vi "Boiler.vi"(8 "error in":errorcluster, 9 "Boiler Configuration":T2, 10 "Notifiers":T1, 11 "Message Queues":T3) -> (0 "error out":errorcluster)   [LabVIEW 2015, in "Boiler.lvlib"]
doc: "This module simulates the behavior of a boiler. It receives a command from the boiler controller, executes, and then notifies the boiler controller that it has completed the operation."
uses:
  Boiler.lvlib
  support/Message Queue/All Message Queues.ctl
  support/Message Queue/Message Cluster.ctl
  Boiler Configuration.ctl
  support/Notifiers/Notifiers.ctl
  Boiler Data.ctl
  Boiler UI Data.ctl
  Boiler References.ctl
  <vilib>/Utility/error.llb/Error Cluster From Error Code.vi
  <vilib>/ErrorRing/Error Ring.xnode
  support/Message Queue/Message Queue.lvlib
panel:
  out "Pilot Flame Level (%)":u32(knob) scale=0.0..100.0
  out "Fuel Level (%)":u32(slide) scale=0.0..100.0
  in  "Simulate Failure":bool
  out "Forced Draft Fan":bool
  out "Pilot":bool
  out "Pilot Gas":bool
  out "Primary Fan":bool
  out "Run Interlock":bool
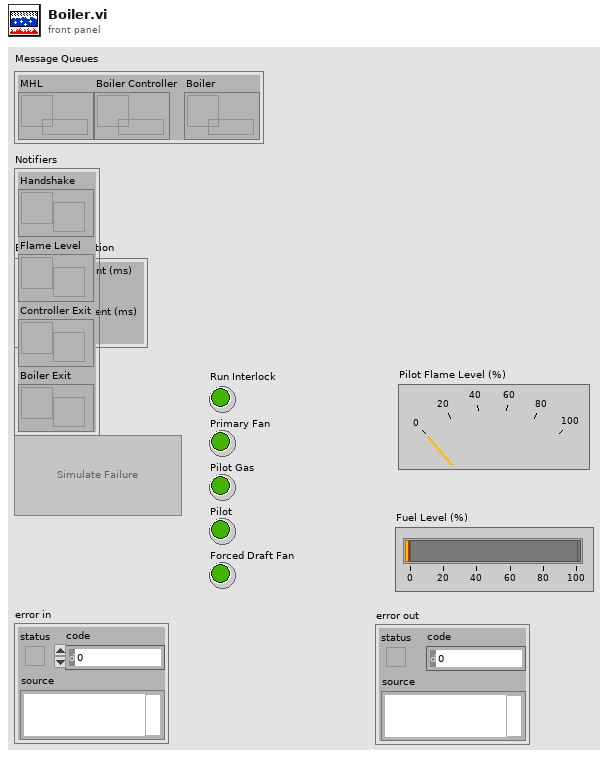
[diagram p1: front panel]
types:
  T1 = typedef "Notifiers.ctl" = cluster{"Handshake":refnum<notifier>, "Flame Level":refnum<notifier>, "Controller Exit":refnum<notifier>, "Boiler Exit":refnum<notifier>}
  T2 = typedef "Boiler.lvlib/Boiler Configuration.ctl" = cluster{"Pilot Increment (ms)":u32, "Pilot Decrement (ms)":u32}
  T3 = typedef "Message Queue.lvlib/All Message Queues.ctl" = cluster{"MHL":refnum<queue>, "Boiler Controller":refnum<queue>, "Boiler":refnum<queue>}
  T4 = typedef "Boiler.lvlib/Boiler Data.ctl" = cluster{"Boiler User Interface Data":T5, "Boiler Configuration":T2, "Boiler References":T6}
  T5 = typedef "Boiler.lvlib/Boiler UI Data.ctl" = cluster{"Run Interlock":bool, "Primary Fan":bool, "Pilot Gas":bool, "Pilot":bool, "Forced Draft Fan":bool, "Pilot Flame Level (%)":u32, "Boiler Flame Level (%)":u32}
  T6 = typedef "Boiler.lvlib/Boiler References.ctl" = cluster{"Simulate Failure":refnum<vi>}
  T7 = enum8{"Enabled", "Disabled", "Disabled and Grayed Out"}
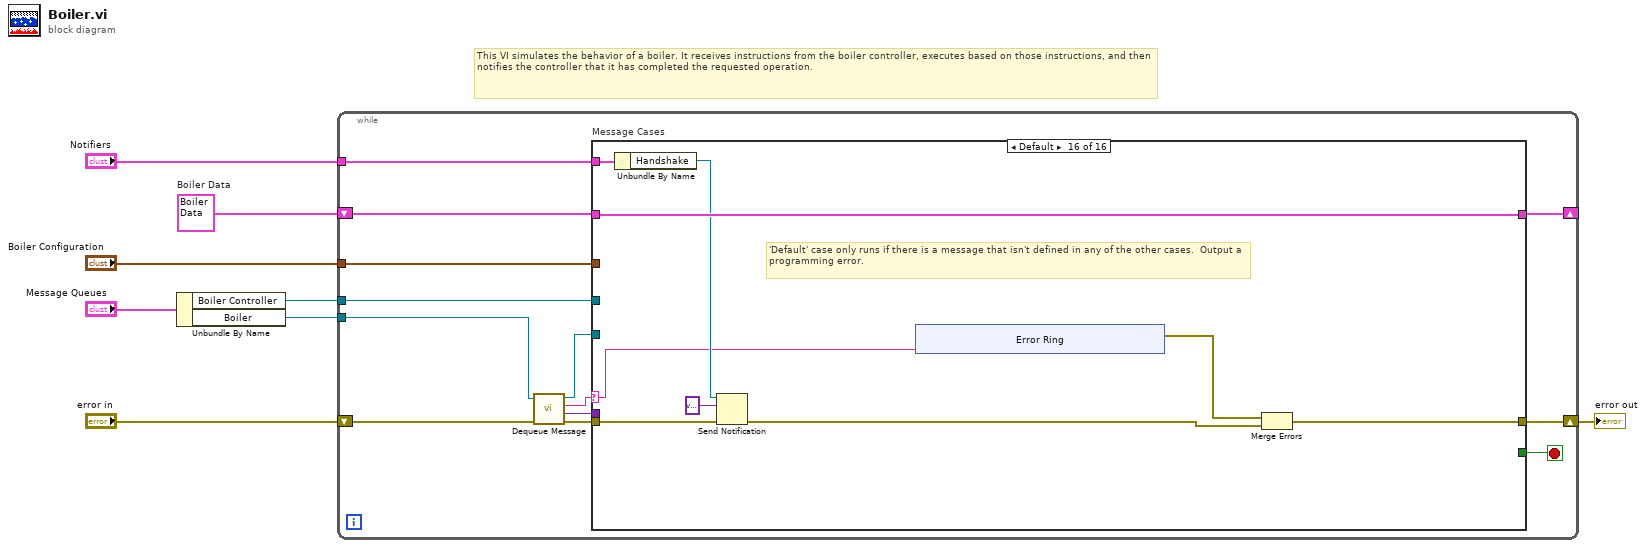
[diagram p0: block diagram]
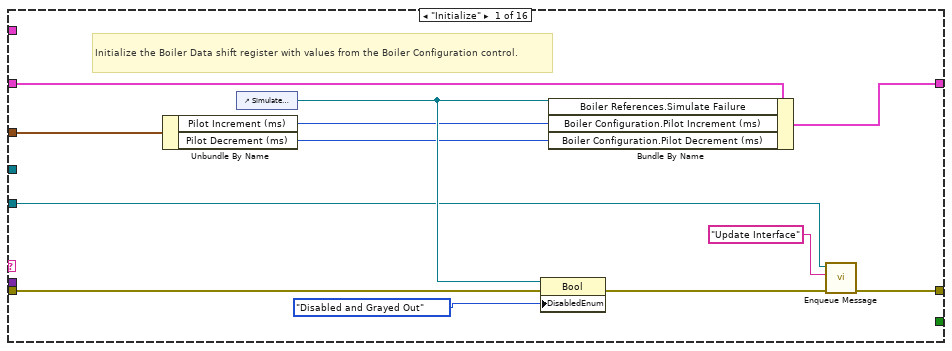
[diagram p2: hidden frame]
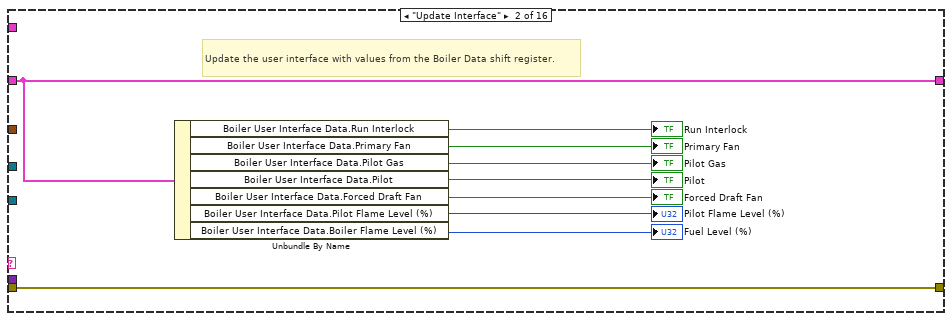
[diagram p3: hidden frame]
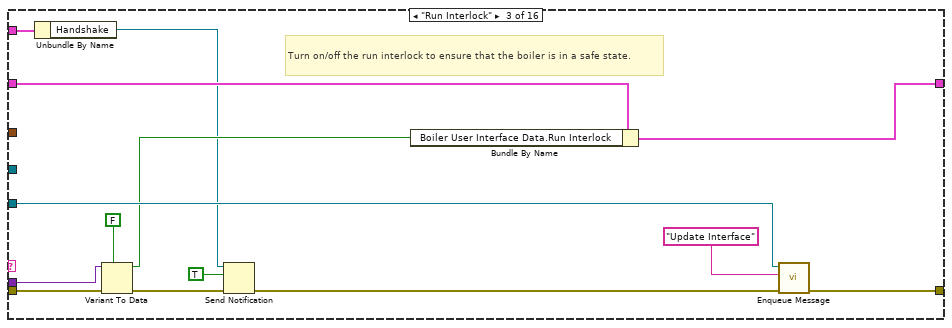
[diagram p4: hidden frame]
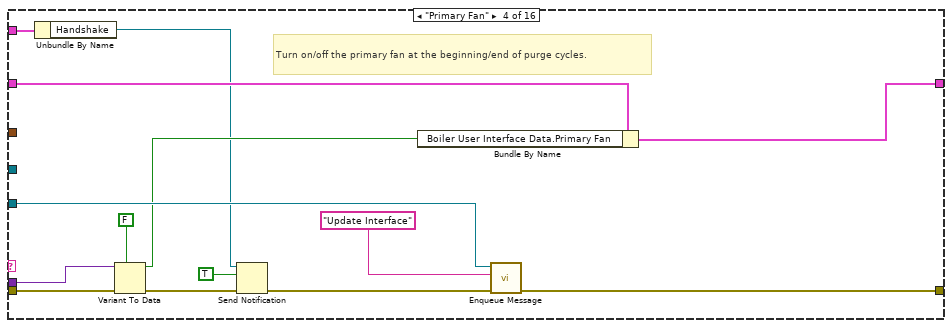
[diagram p5: hidden frame]
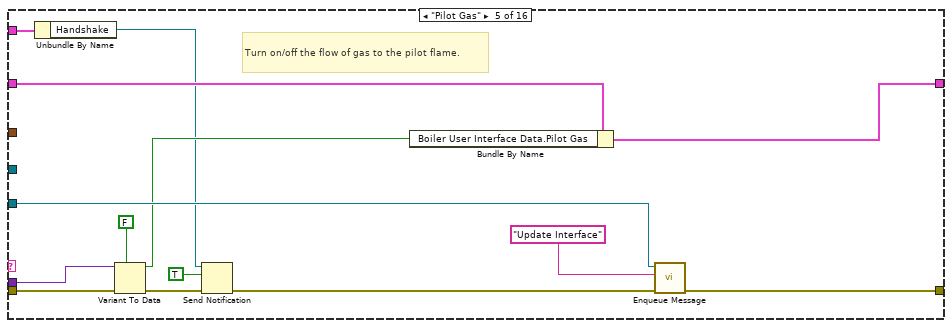
[diagram p6: hidden frame]
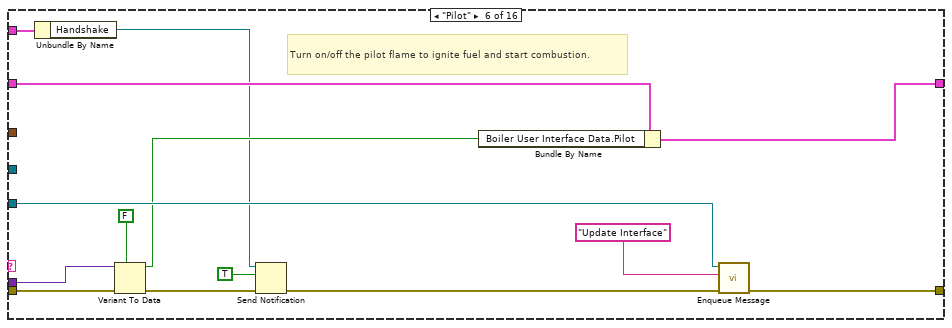
[diagram p7: hidden frame]
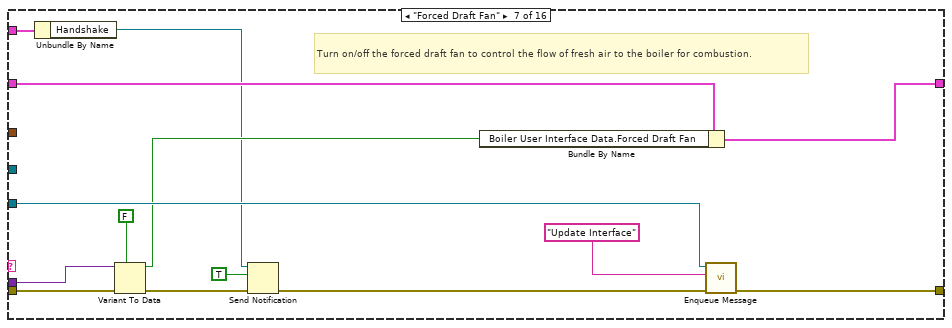
[diagram p8: hidden frame]
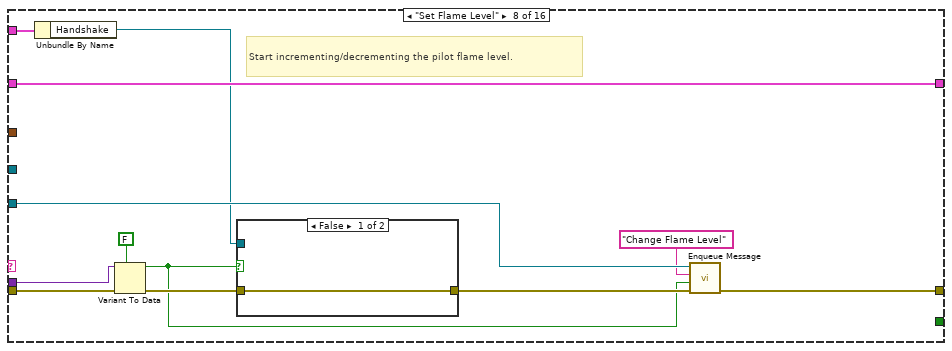
[diagram p9: hidden frame]
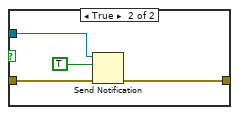
[diagram p10: hidden frame]
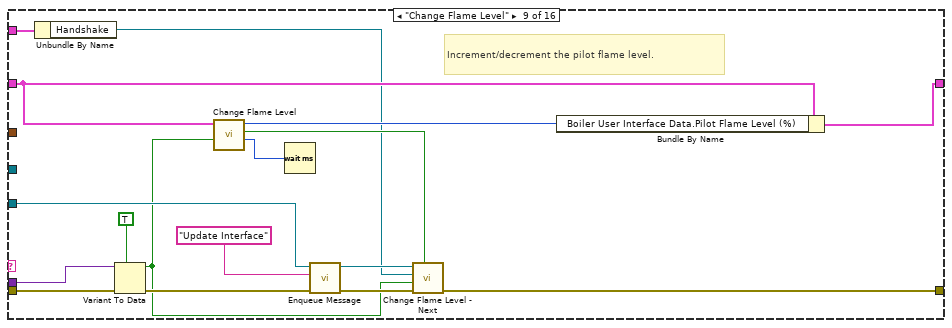
[diagram p11: hidden frame]
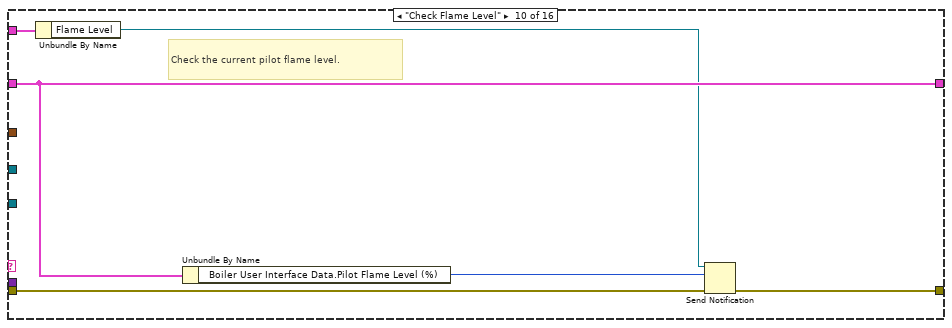
[diagram p12: hidden frame]
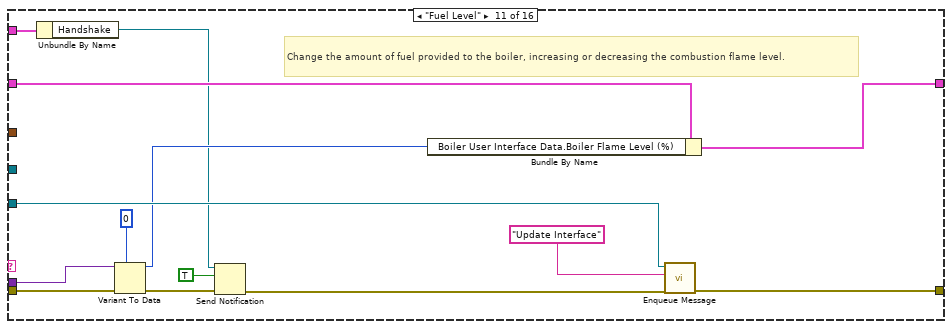
[diagram p13: hidden frame]
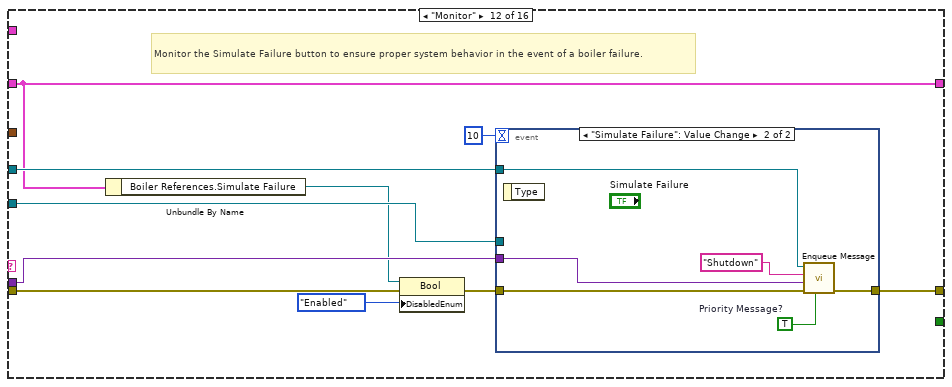
[diagram p14: hidden frame]
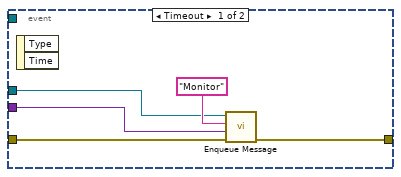
[diagram p15: hidden frame]
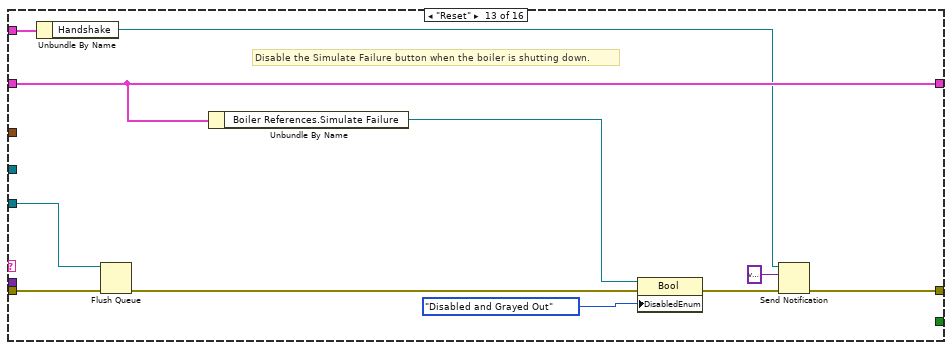
[diagram p16: hidden frame]
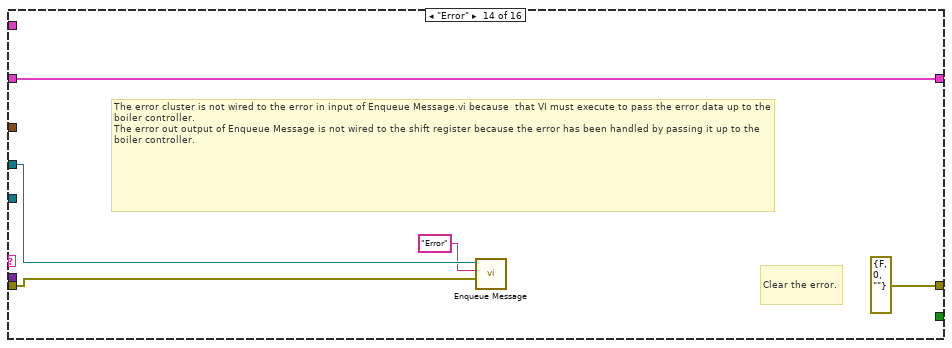
[diagram p17: hidden frame]
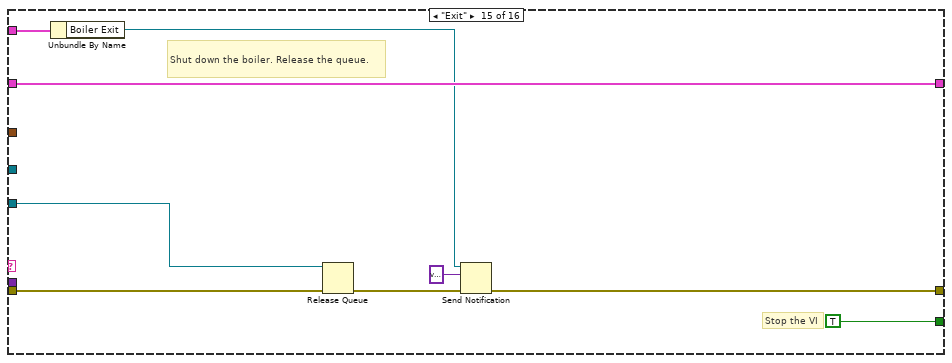
[diagram p18: hidden frame]
diagram:
  w7 = T4 {"Boiler User Interface Data"={"Run Interlock"=FALSE, "Primary Fan"=FALSE, "Pilot Gas"=FALSE, "Pilot"=FALSE, "Forced Draft Fan"=FALSE, "Pilot Flame Level (%)"=0, "Boiler Flame Level (%)"=0}, "Boiler Configuration"={"Pilot Increment (ms)"=0, "Pilot Decrement (ms)"=0}, "Boiler References"={"Simulate Failure"=refnum}}  # Boiler Data
  # "This VI simulates the behavior of a boiler. It receives instructions from the boiler controller, executes based on those instructions, and then notifies the controller that it has completed the requested operation."
  n1 = Unbundle By Name("Message Queues") -> ("Boiler Controller"=w4:refnum<queue>, "Boiler"=w3:refnum<queue>)
  n2 = while {
    tunnel: w3 -> [w12]
    shift-right: [w20] -> _
    shift-left: w7 -> [w21]
    shift-right: [w18] -> w8
    shift-left: "error in" -> [w17]
    tunnel: w4 -> [w11]
    tunnel: "Notifiers" -> [w10]
    tunnel: "Boiler Configuration" -> [w9]
    stop <- w19 stop-if-true
    n3 = call "Dequeue Message.vi"("error in (no error)"=w17, "Message Queue"=w12) -> ("error out"=w16:errorcluster, "Message Data"=w14:variant, "Message"=w15:string, "dup Message Queue"=w13:refnum<queue>)  [unwired: 6 in]
    n4 = case "Message Cases" shown="Default" w15 {
      selector: w15 -> [_ _ _ _ _ _ _ _ _ _ _ _ _ _ _ w213]
      tunnel: w13 -> [w27 _ w56 w66 w80 w94 w108 w122 w143 _ w163 w175 w195 _ w212 _]
      tunnel: w16 -> [w23 w36 w55 w68 w82 w96 w110 w119 w145 w149 w165 w167 w194 w200 w209 w220]
      tunnel: [w28 w36 w47 w60 w74 w88 w102 w123 w134 w152 w156 w168 w192 errorcluster {"status"=FALSE, "code"=0, "source"=""} ("error out") w208 w219] -> w18
      tunnel: w21 -> [w31 w42 w52 w65 w79 w93 w107 w124 w142 w151 w161 w169 w197 w203 w211 w221]
      tunnel: [w32 w42 w49 w64 w78 w92 w105 w124 w141 w151 w159 w169 w197 w203 w211 w221] -> w20
      tunnel: [_ _ _ _ _ _ _ _ _ _ _ _ _ _ TRUE _] -> w19
      tunnel: w14 -> [_ _ w53 w67 w81 w95 w109 w118 w144 _ w164 w173 _ _ _ _]
      tunnel: w11 -> [_ _ _ _ _ _ _ _ _ _ _ w174 _ w202 _ _]
      tunnel: w10 -> [_ _ w45 w59 w73 w87 w101 w114 w133 w150 w155 _ w191 _ w207 w217]
      tunnel: w9 -> [w26 _ _ _ _ _ _ _ _ _ _ _ _ _ _ _]
      frame "Initialize" {
        # "Initialize the Boiler Data shift register with values from the Boiler Configuration control."
        n5 = Unbundle By Name(w26) -> ("Pilot Increment (ms)"=w25:u32, "Pilot Decrement (ms)"=w24:u32)
        n6 = control-ref of="Simulate Failure"() -> (w30:refnum<vi>)
        n7 = property class="Bool"(reference=w30, error in=w23, "DisabledEnum"=T7."Disabled and Grayed Out" ("Disabled")) -> (error out=w22:errorcluster)  [unwired: 1 out]
        n8 = Bundle By Name(cluster=w31, "Boiler References.Simulate Failure"=w30, "Boiler Configuration.Pilot Increment (ms)"=w25, "Boiler Configuration.Pilot Decrement (ms)"=w24) -> (w32:T4)
        n9 = call "Enqueue Message.vi"("error in (no error)"=w22, "Message"="Update Interface", "Message Queue"=w27) -> ("error out"=w28:errorcluster)  [unwired: 7 in, 1 out]
      }
      frame "Update Interface" {
        # "Update the user interface with values from the Boiler Data shift register."
        n10 = Unbundle By Name(w42) -> ("Boiler User Interface Data.Run Interlock"=→"Run Interlock":bool, "Boiler User Interface Data.Primary Fan"=→"Primary Fan":bool, "Boiler User Interface Data.Pilot Gas"=→"Pilot Gas":bool, "Boiler User Interface Data.Pilot"=→"Pilot":bool, "Boiler User Interface Data.Forced Draft Fan"=→"Forced Draft Fan":bool, "Boiler User Interface Data.Pilot Flame Level (%)"=→"Pilot Flame Level (%)":u32, "Boiler User Interface Data.Boiler Flame Level (%)"=→"Fuel Level (%)":u32)
      }
      frame "Run Interlock" {
        # "Turn on/off the run interlock to ensure that the boiler is in a safe state."
        n11 = Unbundle By Name(w45) -> ("Handshake"=w43:refnum<notifier>)
        n12 = Variant To Data(error in=w55, type=FALSE ("Run Interlock"), Variant=w53) -> (data=w51:bool, error out=w48:errorcluster)
        n13 = Send Notification(notification=TRUE, notifier=w43, error in (no error)=w48) -> (error out=w46:errorcluster)  [unwired: 1 out]
        n14 = Bundle By Name(cluster=w52, "Boiler User Interface Data.Run Interlock"=w51) -> (w49:T4)
        n15 = call "Enqueue Message.vi"("error in (no error)"=w46, "Message"="Update Interface", "Message Queue"=w56) -> ("error out"=w47:errorcluster)  [unwired: 7 in, 1 out]
      }
      frame "Primary Fan" {
        # "Turn on/off the primary fan at the beginning/end of purge cycles."
        n16 = Unbundle By Name(w59) -> ("Handshake"=w57:refnum<notifier>)
        n17 = Variant To Data(error in=w68, type=FALSE ("Run Interlock"), Variant=w67) -> (data=w63:bool, error out=w62:errorcluster)
        n18 = Send Notification(notification=TRUE ("Run Interlock"), notifier=w57, error in (no error)=w62) -> (error out=w61:errorcluster)  [unwired: 1 out]
        n19 = Bundle By Name(cluster=w65, "Boiler User Interface Data.Primary Fan"=w63) -> (w64:T4)
        n20 = call "Enqueue Message.vi"("error in (no error)"=w61, "Message"="Update Interface", "Message Queue"=w66) -> ("error out"=w60:errorcluster)  [unwired: 7 in, 1 out]
      }
      frame "Pilot Gas" {
        # "Turn on/off the flow of gas to the pilot flame."
        n21 = Unbundle By Name(w73) -> ("Handshake"=w71:refnum<notifier>)
        n22 = Variant To Data(error in=w82, type=FALSE ("Run Interlock"), Variant=w81) -> (data=w77:bool, error out=w76:errorcluster)
        n23 = Send Notification(notification=TRUE ("Run Interlock"), notifier=w71, error in (no error)=w76) -> (error out=w75:errorcluster)  [unwired: 1 out]
        n24 = Bundle By Name(cluster=w79, "Boiler User Interface Data.Pilot Gas"=w77) -> (w78:T4)
        n25 = call "Enqueue Message.vi"("error in (no error)"=w75, "Message"="Update Interface", "Message Queue"=w80) -> ("error out"=w74:errorcluster)  [unwired: 7 in, 1 out]
      }
      frame "Pilot" {
        # "Turn on/off the pilot flame to ignite fuel and start combustion."
        n26 = Unbundle By Name(w87) -> ("Handshake"=w85:refnum<notifier>)
        n27 = Variant To Data(error in=w96, type=FALSE ("Run Interlock"), Variant=w95) -> (data=w91:bool, error out=w90:errorcluster)
        n28 = Send Notification(notification=TRUE ("Run Interlock"), notifier=w85, error in (no error)=w90) -> (error out=w89:errorcluster)  [unwired: 1 out]
        n29 = Bundle By Name(cluster=w93, "Boiler User Interface Data.Pilot"=w91) -> (w92:T4)
        n30 = call "Enqueue Message.vi"("error in (no error)"=w89, "Message"="Update Interface", "Message Queue"=w94) -> ("error out"=w88:errorcluster)  [unwired: 7 in, 1 out]
      }
      frame "Forced Draft Fan" {
        # "Turn on/off the forced draft fan to control the flow of fresh air to the boiler for combustion."
        n31 = Unbundle By Name(w101) -> ("Handshake"=w99:refnum<notifier>)
        n32 = Variant To Data(error in=w110, type=FALSE ("Run Interlock"), Variant=w109) -> (data=w106:bool, error out=w104:errorcluster)
        n33 = Send Notification(notification=TRUE ("Run Interlock"), notifier=w99, error in (no error)=w104) -> (error out=w103:errorcluster)  [unwired: 1 out]
        n34 = Bundle By Name(cluster=w107, "Boiler User Interface Data.Forced Draft Fan"=w106) -> (w105:T4)
        n35 = call "Enqueue Message.vi"("error in (no error)"=w103, "Message"="Update Interface", "Message Queue"=w108) -> ("error out"=w102:errorcluster)  [unwired: 7 in, 1 out]
      }
      frame "Set Flame Level" {
        # "Start incrementing/decrementing the pilot flame level."
        n36 = Unbundle By Name(w114) -> ("Handshake"=w113:refnum<notifier>)
        n37 = Variant To Data(error in=w119, type=FALSE ("Run Interlock"), Variant=w118) -> (data=w115:bool, error out=w117:errorcluster)
        n38 = case shown="False" w115 {
          tunnel: w117 -> [w125 w129]
          tunnel: [w125 w128] -> w116
          tunnel: w113 -> [_ w126]
          frame False {
          }
          frame True {
            n39 = Send Notification(notification=TRUE ("Run Interlock"), notifier=w126, error in (no error)=w129) -> (error out=w128:errorcluster)  [unwired: 1 out]
          }
        }
        n40 = call "Enqueue Message.vi"("error in (no error)"=w116, "Message Data"=w115, "Message"="Change Flame Level", "Message Queue"=w122) -> ("error out"=w123:errorcluster)  [unwired: 6 in, 1 out]
      }
      frame "Change Flame Level" {
        # "Increment/decrement the pilot flame level."
        n41 = Unbundle By Name(w133) -> ("Handshake"=w131:refnum<notifier>)
        n42 = Variant To Data(error in=w145, type=TRUE, Variant=w144) -> (data=w130:bool, error out=w137:errorcluster)
        n43 = call "Change Flame Level.vi"("Increment?"=w130, "Boiler Data"=w142) -> ("Time Increment"=w138:u32, "Limit?"=w132:bool, "Flame Level"=w139:u32)  [unwired: 7 in]
        n44 = Wait (ms)(milliseconds to wait=w138) -> ()  [unwired: 1 out]
        n45 = call "Enqueue Message.vi"("error in (no error)"=w137, "Message"="Update Interface", "Message Queue"=w143) -> ("error out"=w135:errorcluster, "dup Message Queue"=w136:refnum<queue>)  [unwired: 7 in]
        n46 = call "Change Flame Level - Next.vi"("Limit?"=w132, "error in"=w135, "Increment?"=w130, "Handshake"=w131, "Boiler Queue in"=w136) -> ("error out"=w134:errorcluster)  [unwired: 6 in]
        n47 = Bundle By Name(cluster=w142, "Boiler User Interface Data.Pilot Flame Level (%)"=w139) -> (w141:T4)
      }
      frame "Check Flame Level" {
        # "Check the current pilot flame level."
        n48 = Unbundle By Name(w150) -> ("Flame Level"=w147:refnum<notifier>)
        n49 = Unbundle By Name(w151) -> ("Boiler User Interface Data.Pilot Flame Level (%)"=w148:u32)
        n50 = Send Notification(notification=w148, notifier=w147, error in (no error)=w149) -> (error out=w152:errorcluster)  [unwired: 1 out]
      }
      frame "Fuel Level" {
        # "Change the amount of fuel provided to the boiler, increasing or decreasing the combustion flame level."
        n51 = Unbundle By Name(w155) -> ("Handshake"=w153:refnum<notifier>)
        n52 = Variant To Data(error in=w165, type=u32 0, Variant=w164) -> (data=w160:u32, error out=w158:errorcluster)
        n53 = Send Notification(notification=TRUE ("Run Interlock"), notifier=w153, error in (no error)=w158) -> (error out=w157:errorcluster)  [unwired: 1 out]
        n54 = Bundle By Name(cluster=w161, "Boiler User Interface Data.Boiler Flame Level (%)"=w160) -> (w159:T4)
        n55 = call "Enqueue Message.vi"("error in (no error)"=w157, "Message"="Update Interface", "Message Queue"=w163) -> ("error out"=w156:errorcluster)  [unwired: 7 in, 1 out]
      }
      frame "Monitor" {
        # "Monitor the Simulate Failure button to ensure proper system behavior in the event of a boiler failure."
        n56 = Unbundle By Name(w169) -> ("Boiler References.Simulate Failure"=w172:refnum<vi>)
        n57 = property class="Bool"(reference=w172, error in=w167, "DisabledEnum"=T7."Enabled" ("Disabled")) -> (error out=w170:errorcluster)  [unwired: 1 out]
        n58 = event shown="[1] \"Simulate Failure\": Value Change" {
          selector: _ -> [_ _]
          dyn-events: _ -> [_ _]
          timeout: 10 -> [_ _]
          tunnel: w170 -> [w180 w184]
          tunnel: [w179 w185] -> w168
          tunnel: w175 -> [w178 _]
          tunnel: w174 -> [_ w187]
          tunnel: w173 -> [w177 w183]
          event Timeout {
            n59 = event-data() -> ()  [unwired: 1 in, 2 out]
            n60 = call "Enqueue Message.vi"("error in (no error)"=w180, "Message Data"=w177, "Message"="Monitor", "Message Queue"=w178) -> ("error out"=w179:errorcluster)  [unwired: 6 in, 1 out]
          }
          event "Simulate Failure": Value Change {
            w182 = TRUE  # Priority Message?
            n61 = event-data() -> ()  [unwired: 1 in, 1 out]
            n62 = call "Enqueue Message.vi"("Priority Message? (F)"=w182, "error in (no error)"=w184, "Message Data"=w183, "Message"="Shutdown", "Message Queue"=w187) -> ("error out"=w185:errorcluster)  [unwired: 5 in, 1 out]
          }
        }
      }
      frame "Reset" {
        # "Disable the Simulate Failure button when the boiler is shutting down."
        n63 = Unbundle By Name(w191) -> ("Handshake"=w190:refnum<notifier>)
        n64 = Flush Queue(queue=w195, error in (no error)=w194) -> (error out=w188:errorcluster)  [unwired: 2 out]
        n65 = Unbundle By Name(w197) -> ("Boiler References.Simulate Failure"=w196:refnum<vi>)
        n66 = property class="Bool"(reference=w196, error in=w188, "DisabledEnum"=T7."Disabled and Grayed Out" ("Disabled")) -> (error out=w193:errorcluster)  [unwired: 1 out]
        n67 = Send Notification(notification=variant, notifier=w190, error in (no error)=w193) -> (error out=w192:errorcluster)  [unwired: 1 out]
      }
      frame "Error" {
        # "Clear the error."
        # "The error cluster is not wired to the error in input of Enqueue Message.vi because  that VI must execute to pass the error data up to the boiler controller.\nThe error out output of Enqueue Message is not wired to the shift register because the error has been handled by passing it up to the boiler controller."
        n68 = call "Enqueue Message.vi"("Message Data"=w200, "Message"="Error", "Message Queue"=w202) -> ()  [unwired: 7 in, 2 out]
      }
      frame "Exit" {
        # "Shut down the boiler. Release the queue."
        # "Stop the VI"
        n69 = Unbundle By Name(w207) -> ("Boiler Exit"=w205:refnum<notifier>)
        n70 = Release Queue(queue=w212, error in (no error)=w209) -> (error out=w206:errorcluster)  [unwired: 1 in, 2 out]
        n71 = Send Notification(notification=variant, notifier=w205, error in (no error)=w206) -> (error out=w208:errorcluster)  [unwired: 1 out]
      }
      frame Default {
        # "'Default' case only runs if there is a message that isn't defined in any of the other cases.  Output a programming error."
        n72 = Unbundle By Name(w217) -> ("Handshake"=w216:refnum<notifier>)
        n73 = Send Notification(notification=variant, notifier=w216, error in (no error)=w220) -> (error out=w218:errorcluster)  [unwired: 1 out]
        n74 = xnode "Error Ring"("parameter 0"=w213) -> ("error out"=w214:errorcluster)
        n75 = Merge Errors(w214, w218) -> (w219:errorcluster)
      }
    }
  }
  "error out" <- w8
